vi "case panel.vi"() -> ()   [LabVIEW 2020]
panel:
  out "c":dbl
  in  "b":dbl
  in  "a":dbl
  in  "OK Button":bool
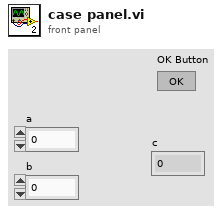
[diagram p1: front panel]
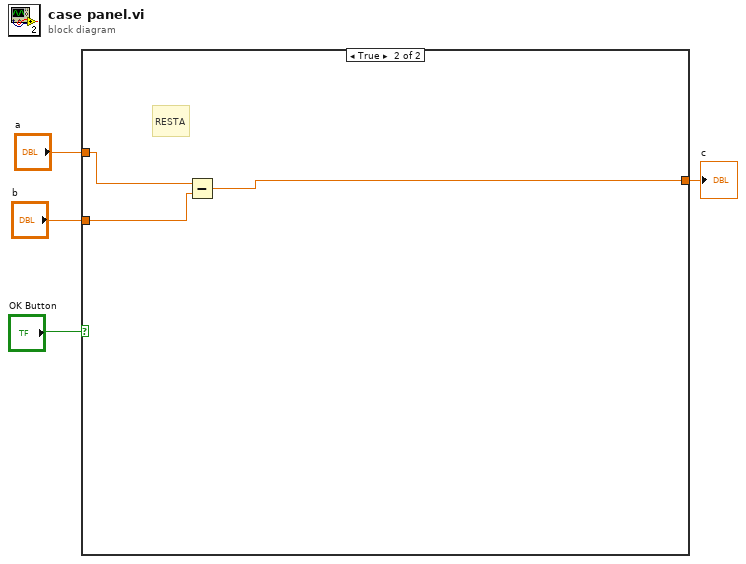
[diagram p0: block diagram]
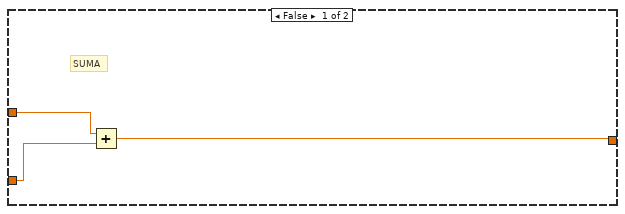
[diagram p2: hidden frame]
diagram:
  n1 = case shown="True" "OK Button" {
    tunnel: "a" -> [w7 w10]
    tunnel: "b" -> [w6 w8]
    tunnel: [w5 w9] -> w1
    frame False {
      # "SUMA"
      n2 = Add(x=w7, y=w6) -> (x+y=w5:dbl)
    }
    frame True {
      # "RESTA"
      n3 = Subtract(x=w10, y=w8) -> (x-y=w9:dbl)
    }
  }
  "c" <- w1
